vi "PH_Trendviewer_Powermeter.PC Set Stat or Trend.vi"(0 "i ref in":refnum<vi>, 1 "Stat or Trend":bool, 5 "error in (no error)":errorcluster) -> (14 "i ref out":refnum<vi>, 19 "error out":errorcluster)   [LabVIEW 2014, in "PH_Trendviewer_Powermeter.lvlib"]
doc: "This VI sets attributes and some GUI elements. It contains the get data to modify / set modified data -vis, handle with care!"
uses:
  PH_Trendviewer_Powermeter.lvlib
  PH_Common/PH_Common.lvlib
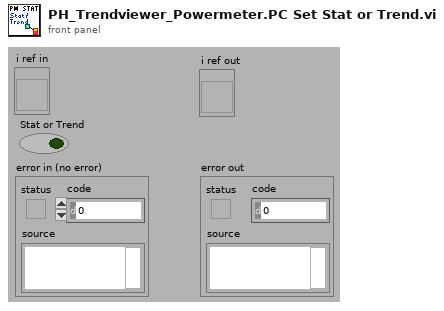
[diagram p1: front panel]
types:
  T1 = typedef "PH_Trendviewer_Powermeter.lvlib/PH_Trendviewer_Powermeter.i attribute.ctl" = cluster{"GUI Refs ":cluster{"Status":refnum<vi>, "Result Graph":refnum<vi>, "Mean Data":refnum<vi>, "Std Dev Data":refnum<vi>, "Dummy Mean":refnum<vi>, "Dummy Std Dev":refnum<vi>, "Export Data":refnum<vi>, "Stat or Trend":refnum<vi>, "Delete":refnum<vi>, "Powermeter":refnum<vi>, "Start":refnum<vi>}, "Powermeter":string, "Stat or Trend":bool, "Start":bool, "Data":cluster{"Time Stamp":timestamp, "Energy [J]":dbl}[], "Datasets strored":i32, "Dataarray Size":i32}
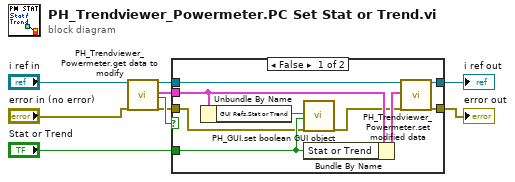
[diagram p0: block diagram]
diagram:
  n1 = call "PH_Trendviewer_Powermeter.get data to modify.vi"("i ref in"="i ref in", "error in (no error)"="error in (no error)") -> ("i ref out"=w4:refnum<vi>, "i attribute"=w8:T1, "timed out"=w7:bool, "error out"=w3:errorcluster)  [unwired: 14 in]
  n2 = case shown="False" w7 {
    tunnel: w3 -> [w10 w19]
    tunnel: w4 -> [w18 w20]
    tunnel: [w17 w20] -> w5
    tunnel: [w16 w19] -> w6
    tunnel: w8 -> [w14 _]
    tunnel: "Stat or Trend" -> [w11 _]
    frame False {
      n3 = Unbundle By Name(w14) -> ("GUI Refs.Stat or Trend"=w12:refnum<vi>)
      n4 = call "PH_GUI.set boolean GUI object.vi"("Boolean Knob GUI Ref"=w12, "Value"=w11, "error in (no error)"=w10) -> ("error out"=w13:errorcluster)  [unwired: 16 in]
      n5 = Bundle By Name(cluster=w14, "Stat or Trend"=w11) -> (w15:T1)
      n6 = call "PH_Trendviewer_Powermeter.set modified data.vi"("i ref in"=w18, "i attribute"=w15, "error in (no error)"=w13) -> ("i ref out"=w17:refnum<vi>, "error out"=w16:errorcluster)  [unwired: 15 in]
    }
    frame True {
    }
  }
  "error out" <- w6
  "i ref out" <- w5
